vi "Define Suite.vi"(5 "Banana Peels":refnum<class "BananaPeel.lvclass">[](array[class]), 7 "Test Report (optional)":refnum<class "Test Report.lvclass">, 8 "error in":errorcluster, 10 "Interactive":bool, 11 "Label (VI Title)":string) -> (0 "error out":errorcluster, 2 "Properties.Suite":refnum<class "Properties.Suite.lvclass">, 3 "Platano":refnum<class "Platano.CarayaTestSuite.lvclass">)   [LabVIEW 2021, in "Banana.Caraya.lvlib" / "Platano.CarayaTestSuite.lvclass"]
uses:
  Banana.Caraya/Platano.CarayaTestSuite/Platano.CarayaTestSuite.lvclass
  <vilib>/addons/_JKI Toolkits/Caraya/classes/Properties.Suite/Properties.Suite.lvclass
  C:/Repositories/LVOS/Bananas/lv-src/Bananas/Platano/Platano.lvclass
  <vilib>/addons/_JKI Toolkits/Caraya/classes/Test Report/Test Report.lvclass
  BananaPeel/BananaPeel.lvclass
  Banana/Banana.lvclass/Banana.ctl
  DefineSuite/DefineSuite.lvclass/DefineSuite.ctl
  DefineSuite/Write Interactive.vi
  <vilib>/LabVIEW Open Source Project/Data Manipulation/Variant/Variant_SetName.vi
  <vilib>/LabVIEW Open Source Project/Data Manipulation/Variant/Variant_BuildClusterFromElementArray.vi
  Banana/Read Ephemerals.vi
  <vilib>/LabVIEW Open Source Project/Data Manipulation/Variant/Variant_EmptyCluster.vi
  DefineSuite/DefineSuite.lvclass
  C:/Repositories/LVOS/Bananas/lv-src/Bananas/BananaPeel/BananaPeel.lvclass
  <vilib>/addons/_JKI Toolkits/Caraya/classes/Test Suite/Define Test Suite (Default).vi
  <vilib>/LabVIEW Open Source Project/Data Manipulation/Variant/Variant_ListElements.vi
  <vilib>/LabVIEW Open Source Project/Data Manipulation/TypeDescriptor/TypeDescriptor_SetName.vi
  <vilib>/Utility/GetType.llb/TD_Create Cluster.vi
  DefineTest/DefineTest.lvclass
  DestroySuite/DestroySuite.lvclass
  Banana/Banana.lvclass
  Platano/Platano.lvclass
  <vilib>/addons/_JKI Toolkits/Caraya/classes/Test Suite/Test Suite.lvclass
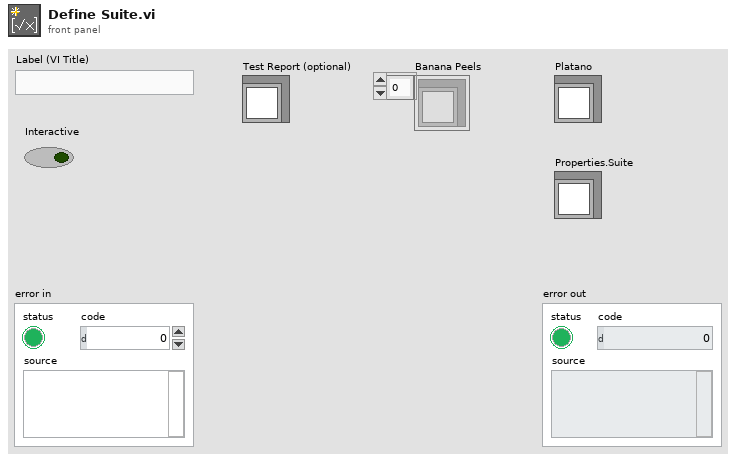
[diagram p1: front panel]
types:
  T1 = typedef "Bananas.lvlib/Test Strategies -- cluster.ctl" = cluster{"DefineTest":refnum<class "DefineTest.lvclass">, "DefineSuite":refnum<class "DefineSuite.lvclass">, "DestroySuite":refnum<class "DestroySuite.lvclass">}
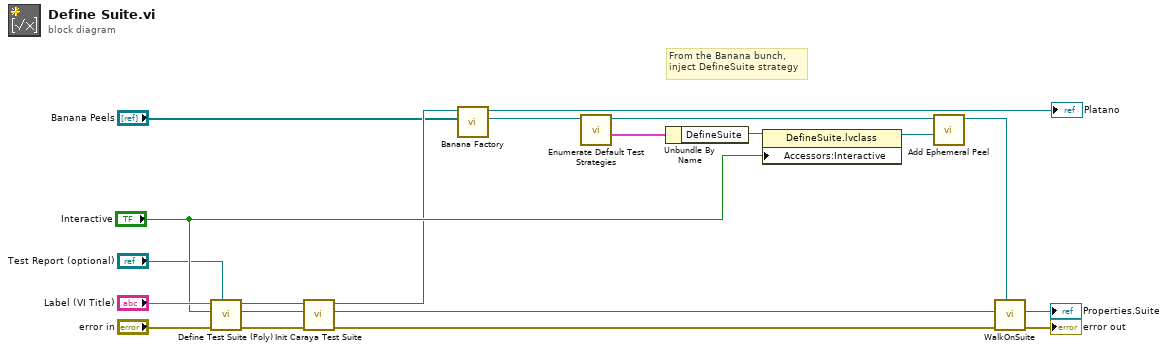
[diagram p0: block diagram]
diagram:
  # "From the Banana bunch,\ninject DefineSuite strategy"
  n1 = call-poly <vilib>:"Define Test Suite (Poly).vi"("Test Report (optional)"="Test Report (optional)", "error in (no error)"="error in", "Interactive"="Interactive", "Label (VI Title)"="Label (VI Title)") -> ("error out"=w9:errorcluster, "Properties.Suite"=w7:refnum<class "Properties.Suite.lvclass">, "Test Suite"=w11:refnum<class "Test Suite.lvclass">)  [unwired: 5 in]
  n2 = call "Init Caraya Test Suite.vi"("error in (no error)"=w9, "Properties.Suite"=w7, "TestSuite"=w11) -> ("error out"=w8:errorcluster, "Properties.Suite dup"=w3:refnum<class "Properties.Suite.lvclass">, "Platano.CarayaTestSuite out"=w6:refnum<class "Platano.CarayaTestSuite.lvclass">)  [unwired: 6 in]
  n3 = call "Banana Factory.vi"("Peels"="Banana Peels", "Platano"=w6) -> ("Banana"=w2:refnum<class "Banana.lvclass">, "Platano dup"=→"Platano":refnum<class "Platano.CarayaTestSuite.lvclass">)  [unwired: 8 in]
  n4 = call "Enumerate Default Test Strategies.vi"("Banana"=w2) -> ("Strategies"=w20:T1, "Banana"=w19:refnum<class "Banana.lvclass">)  [unwired: 9 in]
  n5 = Unbundle By Name(w20) -> ("DefineSuite"=w14:refnum<class "DefineSuite.lvclass">)
  n6 = property class="DefineSuite.lvclass"(reference=w14, "Accessors:Interactive"="Interactive") -> (reference out=w13:refnum<class "DefineSuite.lvclass">)  [unwired: 1 in, 1 out]
  n7 = call "Add Ephemeral Peel.vi"("BananaPeel"=w13, "Banana"=w19) -> ("Banana"=w10:refnum<class "Banana.lvclass">)  [unwired: 9 in]
  n8 = call "WalkOnSuite.vi"("Banana"=w10, "error in (no error)"=w8, "Properties.Suite"=w3) -> ("error out"=→"error out":errorcluster, "Properties.Suite out"=→"Properties.Suite":refnum<class "Properties.Suite.lvclass">)  [unwired: 7 in]
